vi "Color Picker Dialog.vi"(1 "Color in (Unchanged)":u32(colorbox)=16777222) -> (0 "Selected Color":u32(colorbox))   [LabVIEW 2021, in "Image.lvlib"]
uses:
  Image.lvlib
panel:
  in  "Cancel":bool
  in  "OK":bool
  in  "Click & Select Color ---->":u32(colorbox)
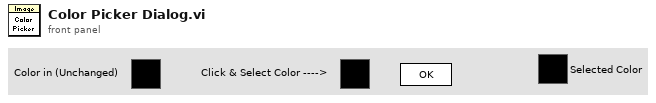
[diagram p1: front panel]
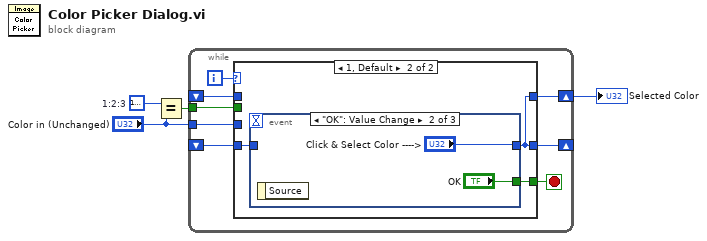
[diagram p0: block diagram]
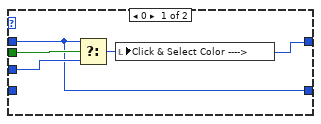
[diagram p2: hidden frame]
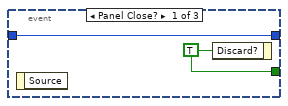
[diagram p3: hidden frame]
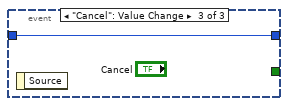
[diagram p4: hidden frame]
diagram:
  w3 = u32 16777222  # 1:2:3
  n1 = Equal?(x=w3, y="Color in (Unchanged)") -> (x = y?=w4:bool)
  n2 = while {
    tunnel: w4 -> [w9]
    shift-right: [w11] -> w1
    shift-left: _ -> [w8]
    tunnel: "Color in (Unchanged)" -> [w7]
    shift-right: [w6] -> _
    shift-left: _ -> [w5]
    i -> [w10]
    stop <- w12 stop-if-true
    n3 = case shown="1, Default" w10 {
      tunnel: [_ w19] -> w12
      tunnel: [w15 w17] -> w11
      tunnel: w9 -> [w16 _]
      tunnel: w8 -> [w13 _]
      tunnel: w7 -> [w14 _]
      tunnel: [w13 w17] -> w6
      tunnel: w5 -> [_ w18]
      frame 0 {
        n4 = Select(t=w13, s=w16, f=w14) -> (s? t:f=w15:u32)
        n5 = local write "Click & Select Color ---->"(w15) -> ()
      }
      frame 1, Default {
        n6 = event shown="[1] \"OK\": Value Change" {
          selector: _ -> [_ _ _]
          dyn-events: _ -> [_ _ _]
          timeout: _ -> [_ _ _]
          tunnel: [w21 "OK" _] -> w19
          tunnel: w18 -> [w20 _ w24]
          tunnel: [w20 "Click & Select Color ---->" w24] -> w17
          event Panel Close? {
            w21 = TRUE ("Discard?")
            n7 = event-data() -> ()  [unwired: 1 in, 1 out]
            n8 = event-data("Discard?"=w21) -> ()  [unwired: 1 in, 1 out]
          }
          event "OK": Value Change {
            n9 = event-data() -> ()  [unwired: 1 in, 1 out]
          }
          event "Cancel": Value Change {
            n10 = event-data() -> ()  [unwired: 1 in, 1 out]
          }
        }
      }
    }
  }
  "Selected Color" <- w1
